vi "Example.vi"() -> ()   [LabVIEW 2014]
doc: "Use this template to build a producer/consumer design pattern with events to produce queue items. Use this design pattern instead of the User Interface Event Handler pattern for user interfaces when you want to execute code asynchronously in response to an event without slowing the user interface responsiveness."
uses:
  TypeDef.ctl
  <vilib>/DAQmx/create/channels.llb/DAQmx Create Channel (AI-Voltage-Basic).vi
  <vilib>/DAQmx/configure/timing.llb/DAQmx Timing (Sample Clock).vi
  <vilib>/DAQmx/read.llb/DAQmx Read (Analog DBL 1Chan 1Samp).vi
  <vilib>/Utility/file.llb/Write To Spreadsheet File (DBL).vi
panel:
  in  "Start DAQ 2":bool
  in  "Stop DAQ 2":bool
  out "AI 1 Data":dbl[](graph)
  out "AI 0 Data":dbl[](graph)
  in  "Stop Program":bool
  in  "Start DAQ":bool
  in  "Stop DAQ":bool
  # "AI 0"
  # "You can start and stop AI0 and AI1 independent of one another while the program is running.  When you stop a task, a popup will ask you where you want to save the data in an excel file."
  # "AI 1"
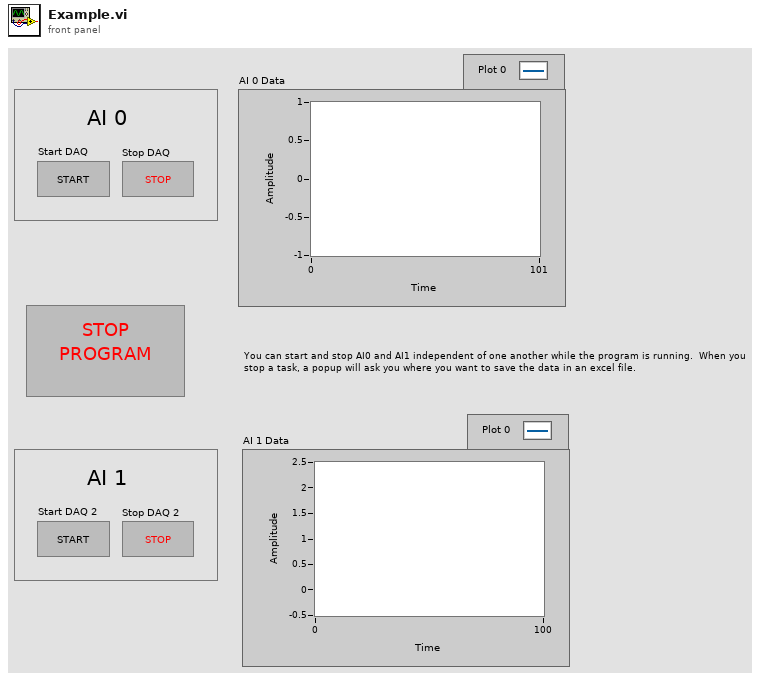
[diagram p1: front panel]
types:
  T1 = typedef "TypeDef.ctl" = enum16{"Idle", "Initialize", "Acquire", "Stop"}
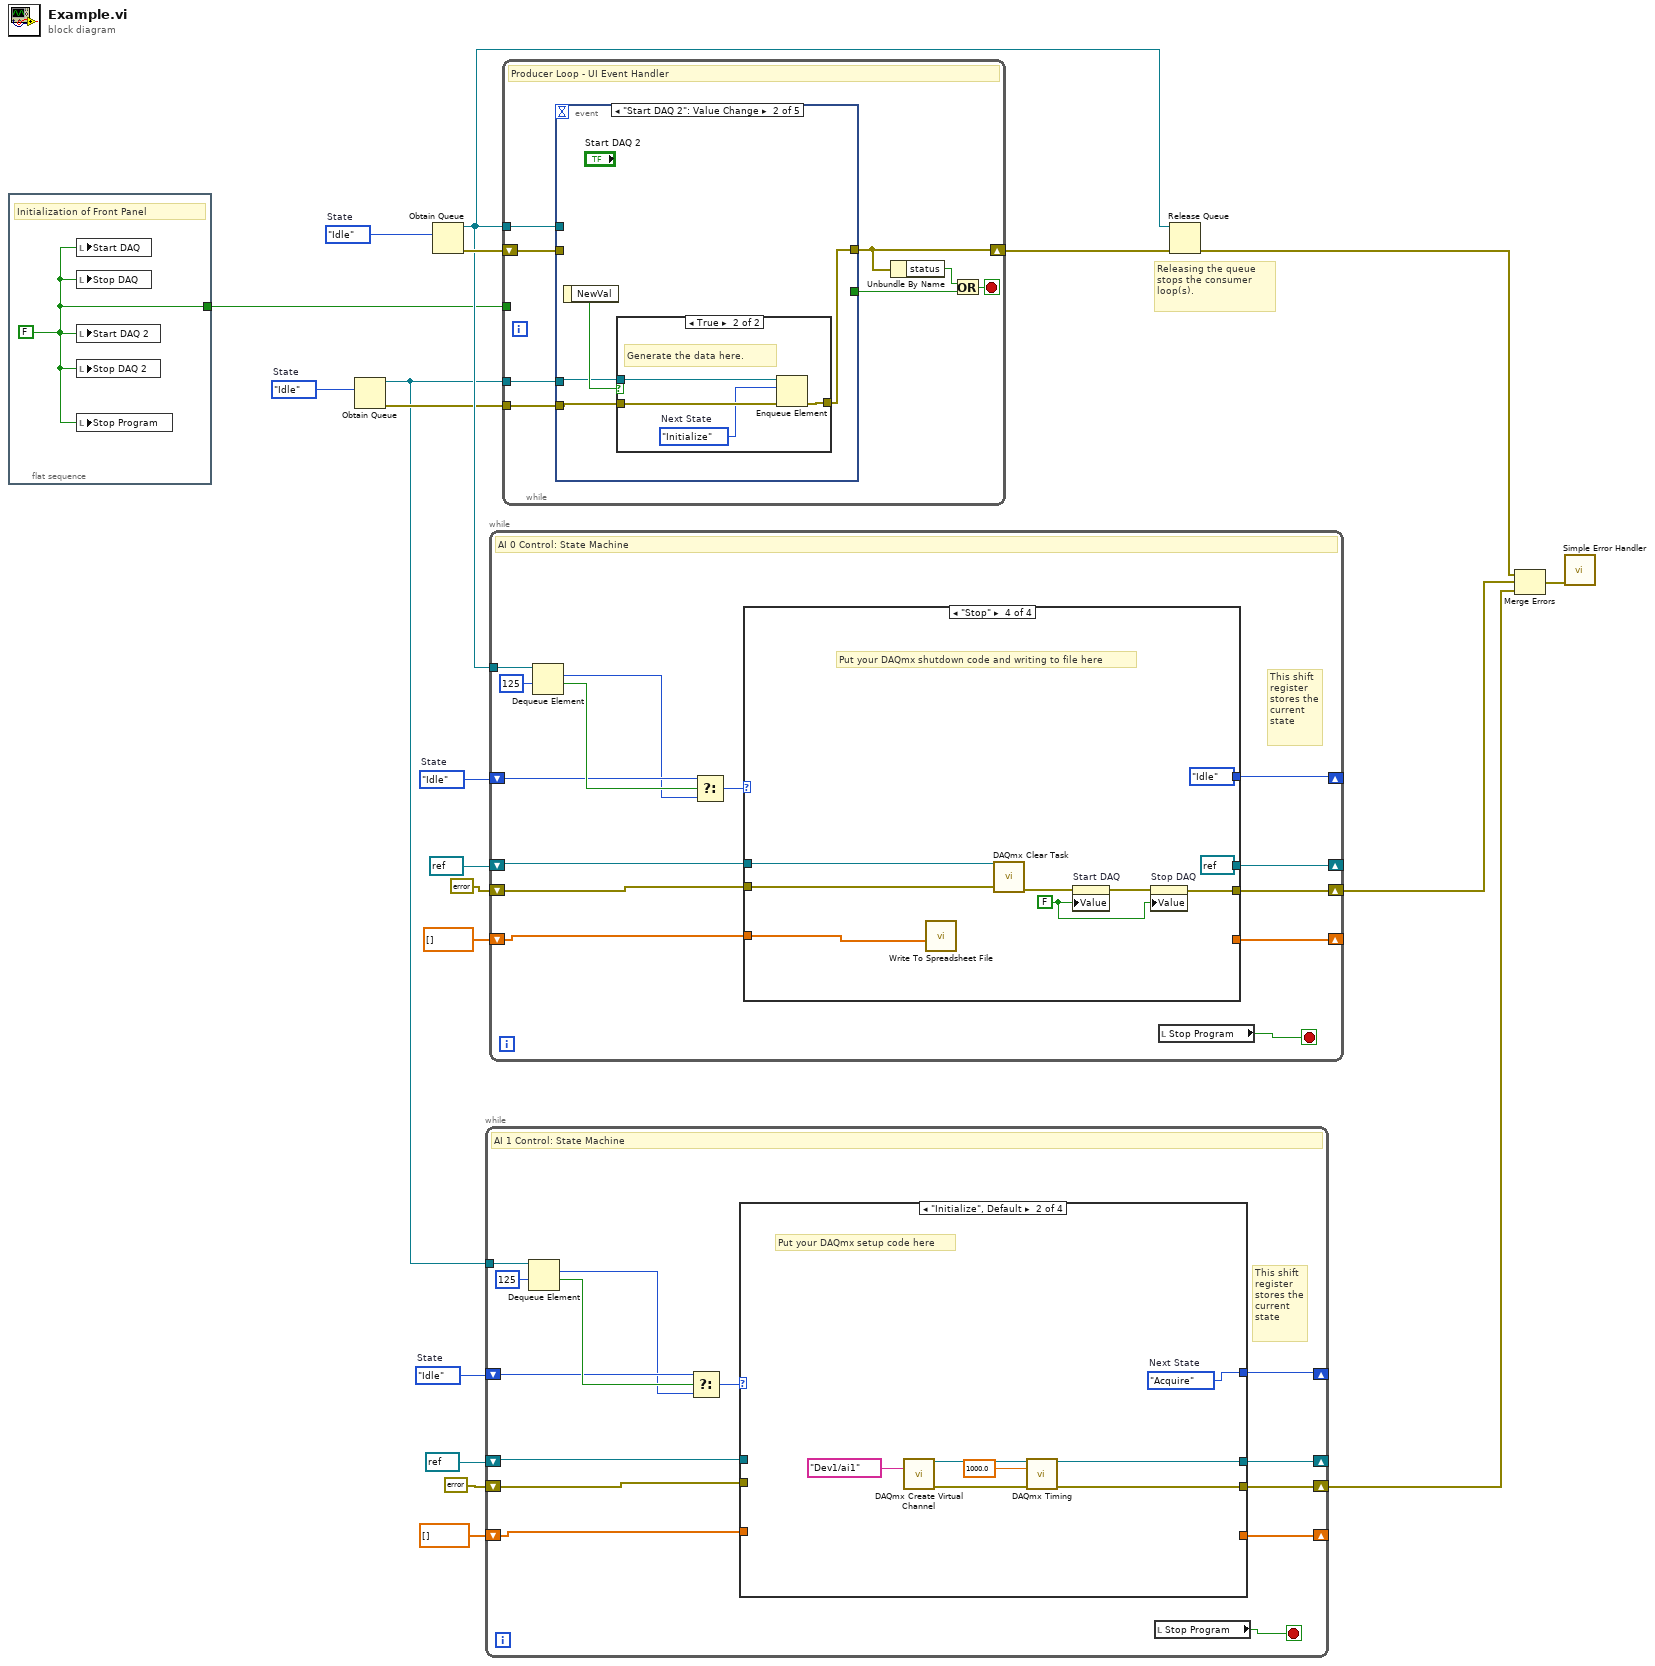
[diagram p0: block diagram]
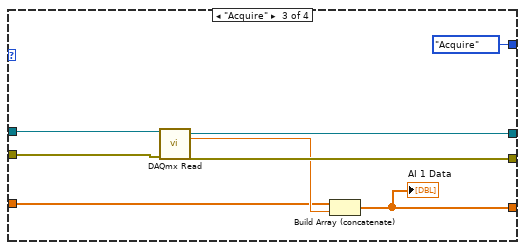
[diagram p3: hidden frame]
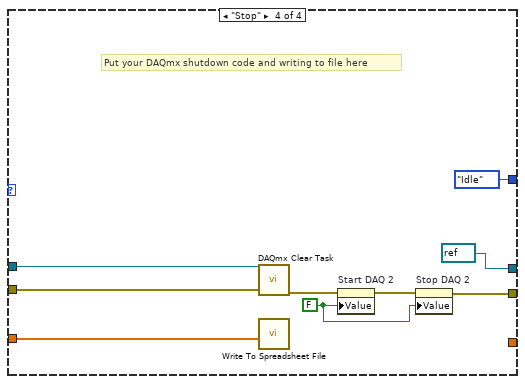
[diagram p4: hidden frame]
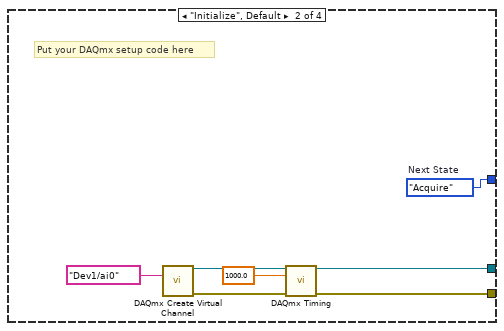
[diagram p6: hidden frame]
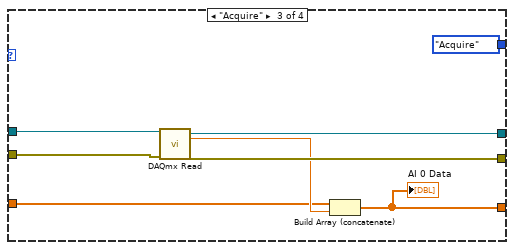
[diagram p7: hidden frame]
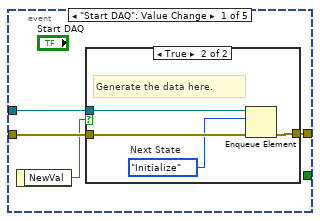
[diagram p8: hidden frame]
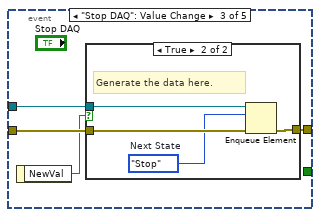
[diagram p11: hidden frame]
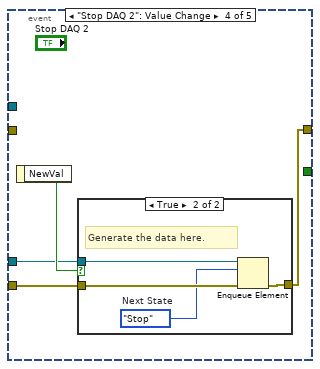
[diagram p13: hidden frame]
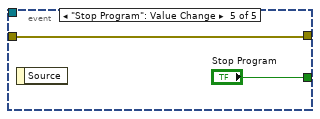
[diagram p15: hidden frame]
diagram:
  w7 = TypeDef."Idle"  # State
  w8 = TypeDef."Idle"  # State
  w16 = TypeDef."Idle"  # State
  w17 = TypeDef."Idle"  # State
  # "Releasing the queue stops the consumer loop(s)."
  n1 = flat-sequence {
    tunnel: [w21] -> w12
    frame #0 {
      w21 = FALSE ("Stop Program")
      # "Initialization of Front Panel"
      n2 = local write "Start DAQ"(w21) -> ()
      n3 = local write "Stop DAQ"(w21) -> ()
      n4 = local write "Start DAQ 2"(w21) -> ()
      n5 = local write "Stop DAQ 2"(w21) -> ()
      n6 = local write "Stop Program"(w21) -> ()
    }
  }
  n7 = Obtain Queue(element data type=w7) -> (queue out=w5:refnum<queue>, error out=w6:errorcluster)  [unwired: 4 in, 1 out]
  n8 = Obtain Queue(element data type=w17) -> (queue out=w18:refnum<queue>, error out=w20:errorcluster)  [unwired: 4 in, 1 out]
  n9 = while {
    shift-right: [w30] -> _
    shift-left: w8 -> [w32]
    shift-right: [w28] -> _
    shift-left: refnum<k21> refnum ("task out") -> [w26]
    shift-right: [w27] -> w4
    shift-left: errorcluster {"status"=FALSE, "code"=0, "source"=""} ("error out") -> [w25]
    shift-right: [w24] -> _
    shift-left: dbl[] [] -> [w23]
    tunnel: w5 -> [w22]
    stop <- w29 stop-if-true
    # "This shift\nregister\nstores the\ncurrent\nstate"
    # "AI 1 Control: State Machine"
    n10 = Dequeue Element(queue=w22, timeout in ms (-1)=125) -> (element=w31:T1, timed out?=w34:bool)  [unwired: 1 in, 2 out]
    n11 = Select(t=w32, s=w34, f=w31) -> (s? t:f=w33:T1)
    n12 = case shown="\"Initialize\", Default" w33 {
      selector: w33 -> [w37 _ _ _]
      tunnel: [w37 w44 TypeDef."Acquire" ("Next State") TypeDef."Idle" ("Next State")] -> w30
      tunnel: [_ w40 w51 refnum<k21> refnum ("task out")] -> w28
      tunnel: [w36 w38 w49 w54] -> w27
      tunnel: w26 -> [_ _ w50 w59]
      tunnel: w25 -> [w36 _ w48 w60]
      tunnel: [_ _ w46 _] -> w24
      tunnel: w23 -> [_ _ w45 w56]
      frame "Idle" {
      }
      frame "Initialize", Default {
        w44 = TypeDef."Acquire"  # Next State
        # "Put your DAQmx setup code here"
        n13 = call-poly <vilib>:"DAQmx Create Virtual Channel.vi"("physical channels"=tag "Dev1/ai1") -> ("task out"=w42:refnum<k21>, "error out"=w39:errorcluster)  [unwired: 13 in]
        n14 = call-poly <vilib>:"DAQmx Timing.vi"("task/channels in"=w42, "rate"=1000.0, "error in"=w39) -> ("task out"=w40:refnum<k21>, "error out"=w38:errorcluster)  [unwired: 11 in]
      }
      frame "Acquire" {
        n15 = call-poly <vilib>:"DAQmx Read.vi"("task/channels in"=w50, "error in"=w48) -> ("task out"=w51:refnum<k21>, "data"=w47:dbl, "error out"=w49:errorcluster)  [unwired: 11 in]
        n16 = Build Array (concatenate)(w45, w47) -> (w46:dbl[])
        "AI 1 Data" <- w46
      }
      frame "Stop" {
        w53 = FALSE ("Start DAQ")
        # "Put your DAQmx shutdown code and writing to file here"
        n17 = call <vilib>:"DAQmx Clear Task.vi"("task in"=w59, "error in"=w60) -> ("error out"=w58:errorcluster)  [unwired: 13 in]
        n18 = call-poly <vilib>:"Write To Spreadsheet File.vi"("1D data"=w56) -> ()  [unwired: 7 in, 1 out]
        n19 = property on="Start DAQ 2" class="Bool (strict)"(error in=w58, "Value"=w53) -> (error out=w55:errorcluster)  [unwired: 1 in, 1 out]
        n20 = property on="Stop DAQ 2" class="Bool (strict)"(error in=w55, "Value"=w53) -> (error out=w54:errorcluster)  [unwired: 1 in, 1 out]
      }
    }
    n21 = local read "Stop Program"() -> (w29:bool)
  }
  n22 = while {
    tunnel: w18 -> [w75]
    shift-right: [w69] -> _
    shift-left: w16 -> [w71]
    shift-right: [w67] -> _
    shift-left: refnum<k21> refnum ("task out") -> [w65]
    shift-right: [w66] -> w3
    shift-left: errorcluster {"status"=FALSE, "code"=0, "source"=""} ("error out") -> [w64]
    shift-right: [w63] -> _
    shift-left: dbl[] [] -> [w62]
    stop <- w68 stop-if-true
    # "This shift\nregister\nstores the\ncurrent\nstate"
    # "AI 0 Control: State Machine"
    n23 = Dequeue Element(queue=w75, timeout in ms (-1)=125) -> (element=w70:T1, timed out?=w73:bool)  [unwired: 1 in, 2 out]
    n24 = Select(t=w71, s=w73, f=w70) -> (s? t:f=w72:T1)
    n25 = case shown="\"Stop\"" w72 {
      selector: w72 -> [w77 _ _ _]
      tunnel: [w77 w84 TypeDef."Acquire" ("Next State") TypeDef."Idle" ("Next State")] -> w69
      tunnel: [_ w80 w91 refnum<k21> refnum ("task out")] -> w67
      tunnel: [w76 w78 w89 w94] -> w66
      tunnel: w65 -> [_ _ w90 w99]
      tunnel: w64 -> [w76 _ w88 w100]
      tunnel: [_ _ w86 _] -> w63
      tunnel: w62 -> [_ _ w85 w96]
      frame "Idle" {
        # "This case is when you are not acquiring data, to prevent you actually having\nto stop the while loop"
      }
      frame "Initialize", Default {
        w84 = TypeDef."Acquire"  # Next State
        # "Put your DAQmx setup code here"
        n26 = call-poly <vilib>:"DAQmx Create Virtual Channel.vi"("physical channels"=tag "Dev1/ai0") -> ("task out"=w82:refnum<k21>, "error out"=w79:errorcluster)  [unwired: 13 in]
        n27 = call-poly <vilib>:"DAQmx Timing.vi"("task/channels in"=w82, "rate"=1000.0, "error in"=w79) -> ("task out"=w80:refnum<k21>, "error out"=w78:errorcluster)  [unwired: 11 in]
      }
      frame "Acquire" {
        n28 = call-poly <vilib>:"DAQmx Read.vi"("task/channels in"=w90, "error in"=w88) -> ("task out"=w91:refnum<k21>, "data"=w87:dbl, "error out"=w89:errorcluster)  [unwired: 11 in]
        n29 = Build Array (concatenate)(w85, w87) -> (w86:dbl[])
        "AI 0 Data" <- w86
      }
      frame "Stop" {
        w93 = FALSE ("Start DAQ")
        # "Put your DAQmx shutdown code and writing to file here"
        n30 = call-poly <vilib>:"Write To Spreadsheet File.vi"("1D data"=w96) -> ()  [unwired: 7 in, 1 out]
        n31 = call <vilib>:"DAQmx Clear Task.vi"("task in"=w99, "error in"=w100) -> ("error out"=w98:errorcluster)  [unwired: 13 in]
        n32 = property on="Start DAQ" class="Bool (strict)"(error in=w98, "Value"=w93) -> (error out=w95:errorcluster)  [unwired: 1 in, 1 out]
        n33 = property on="Stop DAQ" class="Bool (strict)"(error in=w95, "Value"=w93) -> (error out=w94:errorcluster)  [unwired: 1 in, 1 out]
      }
    }
    n34 = local read "Stop Program"() -> (w68:bool)
  }
  n35 = while {
    shift-right: [w105] -> w19
    shift-left: w20 -> [w108]
    tunnel: w18 -> [w109]
    tunnel: w12 -> [_]
    tunnel: w5 -> [w103]
    tunnel: w6 -> [w102]
    stop <- w106 stop-if-true
    # "Producer Loop - UI Event Handler"
    n36 = event shown="[1] \"Start DAQ 2\": Value Change" {
      selector: _ -> [_ _ _ _ _]
      dyn-events: _ -> [_ _ _ _ _]
      timeout: _ -> [_ _ _ _ _]
      tunnel: w109 -> [w113 _ w131 _ _]
      tunnel: w108 -> [w112 _ w130 _ w147]
      tunnel: [w111 w122 w129 w140 w147] -> w105
      tunnel: [_ _ _ _ "Stop Program"] -> w107
      tunnel: w103 -> [_ w120 _ w138 _]
      tunnel: w102 -> [_ w119 _ w137 _]
      event "Start DAQ": Value Change {
        n37 = event-data() -> ("NewVal"=w110:bool)  [unwired: 1 in]
        n38 = case shown="True" w110 {
          tunnel: w113 -> [_ w118]
          tunnel: w112 -> [w114 w117]
          tunnel: [w114 w116] -> w111
          frame False {
          }
          frame True {
            w115 = TypeDef."Initialize"  # Next State
            # "Generate the data here."
            n39 = Enqueue Element(queue=w118, element=w115, error in (no error)=w117) -> (error out=w116:errorcluster)  [unwired: 1 in, 2 out]
          }
        }
      }
      event "Start DAQ 2": Value Change {
        n40 = event-data() -> ("NewVal"=w121:bool)  [unwired: 1 in]
        n41 = case shown="True" w121 {
          tunnel: w120 -> [_ w127]
          tunnel: w119 -> [w123 w126]
          tunnel: [w123 w125] -> w122
          frame False {
          }
          frame True {
            w124 = TypeDef."Initialize"  # Next State
            # "Generate the data here."
            n42 = Enqueue Element(queue=w127, element=w124, error in (no error)=w126) -> (error out=w125:errorcluster)  [unwired: 1 in, 2 out]
          }
        }
      }
      event "Stop DAQ": Value Change {
        n43 = event-data() -> ("NewVal"=w128:bool)  [unwired: 1 in]
        n44 = case shown="True" w128 {
          tunnel: w131 -> [_ w136]
          tunnel: w130 -> [w132 w135]
          tunnel: [w132 w134] -> w129
          frame False {
          }
          frame True {
            w133 = TypeDef."Stop"  # Next State
            # "Generate the data here."
            n45 = Enqueue Element(queue=w136, element=w133, error in (no error)=w135) -> (error out=w134:errorcluster)  [unwired: 1 in, 2 out]
          }
        }
      }
      event "Stop DAQ 2": Value Change {
        n46 = event-data() -> ("NewVal"=w139:bool)  [unwired: 1 in]
        n47 = case shown="True" w139 {
          tunnel: w138 -> [_ w145]
          tunnel: w137 -> [w141 w144]
          tunnel: [w141 w143] -> w140
          frame False {
          }
          frame True {
            w142 = TypeDef."Stop"  # Next State
            # "Generate the data here."
            n48 = Enqueue Element(queue=w145, element=w142, error in (no error)=w144) -> (error out=w143:errorcluster)  [unwired: 1 in, 2 out]
          }
        }
      }
      event "Stop Program": Value Change {
        n49 = event-data() -> ()  [unwired: 1 in, 1 out]
      }
    }
    n50 = Unbundle By Name(w105) -> ("status"=w104:bool)
    n51 = Or(x=w104, y=w107) -> (x .or. y?=w106:bool)
  }
  n52 = Release Queue(queue=w18, error in (no error)=w19) -> (error out=w2:errorcluster)  [unwired: 1 in, 2 out]
  n53 = Merge Errors(w2, w3, w4) -> (w1:errorcluster)
  n54 = call <vilib>:"Simple Error Handler.vi"("error in (no error)"=w1) -> ()  [unwired: 4 in, 5 out]
